vi "Get.vi"(8 "error in (no error)":errorcluster, 11 "ByRef in":refnum<class "ByRef.lvclass">) -> (0 "error out":errorcluster, 2 "Dummy":i32, 3 "ByRef out":refnum<class "ByRef.lvclass">)   [LabVIEW 2020, in "ByRef.lvclass"]
uses:
  ByRef.lvclass
  ByRef.lvclass/ByRef.ctl
  Private/TypeDef/privateDataDVR.ctl
  Private/TypeDef/privateData.ctl
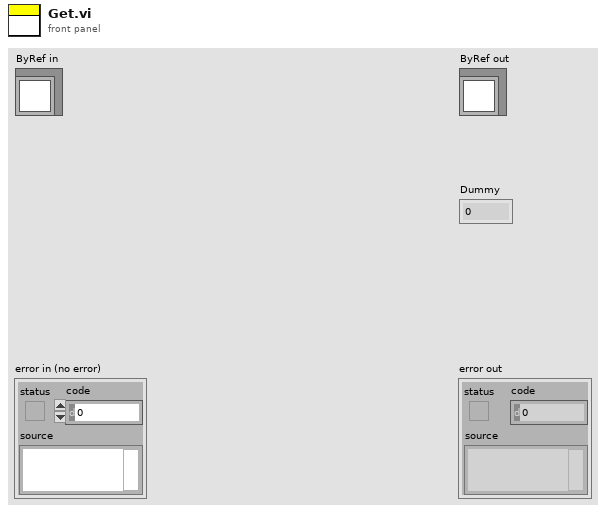
[diagram p1: front panel]
types:
  T1 = typedef "ByRef.lvclass/privateDataDVR.ctl" = refnum<data-value>
  T2 = typedef "ByRef.lvclass/privateData.ctl" = cluster{"Dummy":i32}
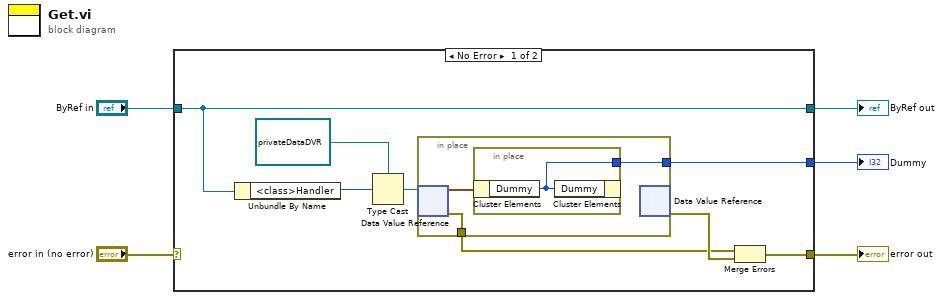
[diagram p0: block diagram]
diagram:
  n1 = case shown="No Error" "error in (no error)" {
    selector: "error in (no error)" -> [_ w19]
    tunnel: [w7 w19] -> w4
    tunnel: [w9 w18] -> w2
    tunnel: "ByRef in" -> [w9 w18]
    tunnel: [w6 _] -> w1
    frame No Error {
      n2 = Unbundle By Name(w9) -> ("<class>Handler"=w11:u32)
      n3 = Type Cast(type=T1 refnum ("privateDataDVR"), x=w11) -> (*(type *) &x=w13:T1)
      n4 = in-place {
        in-place-border: [w15] -> w6
        in-place-border: [w14] -> w10
        n5 = in-place-dvr #1(w13) -> (w16:T2, w14:errorcluster)
        n6 = in-place {
          in-place-border: [w17] -> w15
          n7 = in-place-cluster #2(w16) -> ("Dummy"=w17:i32)
          n8 = in-place-cluster #2("Dummy"=w17) -> ()  [unwired: 1 out]
        }
        n9 = in-place-dvr #1() -> (w12:errorcluster)  [unwired: 1 in, 1 out]
      }
      n10 = Merge Errors(w10, w12) -> (w7:errorcluster)
    }
    frame Error {
    }
  }
  "error out" <- w4
  "ByRef out" <- w2
  "Dummy" <- w1
